vi "Get Linked List Name.vi"(8 "error in (no error)":errorcluster, 10 "Unique ID":string, 11 "Linked List in":refnum<class "Linked List.lvclass">) -> (0 "error out":errorcluster, 1 "I am Root?":bool, 2 "Linked List Name":string, 3 "Linked List out":refnum<class "Linked List.lvclass">)   [LabVIEW 2020, in "Linked Lists.lvlib" / "Linked List.lvclass"]
uses:
  <vilib>/gpm_packages/@cs/linked-list/Source/Linked List/Linked List/Linked List.lvclass
  <vilib>/gpm_packages/@cs/linked-list/Source/Linked List/Linked List Definition/Linked List Definition.lvclass
  <vilib>/gpm_packages/@cs/linked-list/Source/Linked List/Linked List/Linked List.lvclass/Linked List.ctl
  <vilib>/gpm_packages/@cs/lookup-table/Source/LookupTable/LookupTable.lvclass/LookupTable.ctl
  6b1855ba-96a8-42ce-880d-34d98a0d5dd7.vi
  <vilib>/gpm_packages/@cs/lookup-table/Source/LookupTable/Read Table Reference.vi
  6b1855ba-96a8-42ce-880d-34d98a0d5dd7.vi/5a7267ad-595e-4610-9ac2-8bef780848ff.vi
  <vilib>/gpm_packages/@cs/lookup-table/Source/LookupTable/LookupTable.lvclass
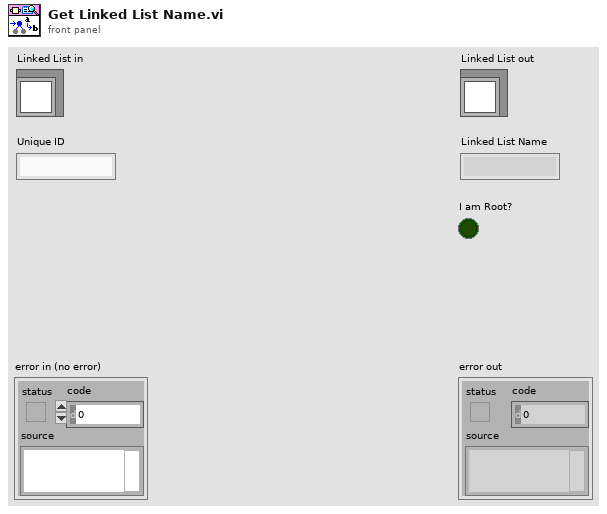
[diagram p1: front panel]
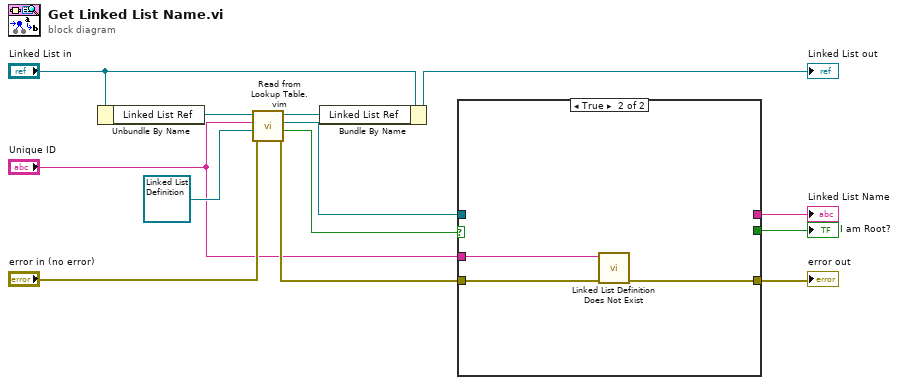
[diagram p0: block diagram]
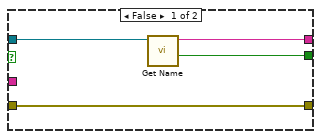
[diagram p2: hidden frame]
diagram:
  n1 = Unbundle By Name("Linked List in") -> ("Linked List Ref"=w13:refnum<data-value>)
  n2 = call "Read from Lookup Table.vim"("error in (no error)"="error in (no error)", "Type"=refnum<class "Linked List Definition.lvclass"> refnum ("Linked List.lvlib:Linked List Definition.lvclass"), "Item Name"="Unique ID", "LookupTable Reference"=w13) -> ("error out"=w5:errorcluster, "Not Found?"=w7:bool, "Value"=w6:refnum<class "Linked List Definition.lvclass">, "LookupTable Reference Out"=w10:refnum<data-value>)  [unwired: 4 in]
  n3 = Bundle By Name(cluster="Linked List in", "Linked List Ref"=w10) -> (→"Linked List out":refnum<class "Linked List.lvclass">)
  n4 = case shown="True" w7 {
    tunnel: w6 -> [w16 _]
    tunnel: w5 -> [w17 w20]
    tunnel: [w17 w19] -> w4
    tunnel: "Unique ID" -> [_ w18]
    tunnel: [w15 _] -> w2
    tunnel: [w14 _] -> w1
    frame False {
      n5 = call <vilib>:"Get Name.vi"("Linked List Definition in"=w16) -> ("I am Root?"=w14:bool, "Name"=w15:string)  [unwired: 8 in, 1 out]
    }
    frame True {
      n6 = call <vilib>:"Linked List Definition Does Not Exist.vi"("Error In"=w20, "Unique ID"=w18) -> ("Error Out"=w19:errorcluster)  [unwired: 9 in]
    }
  }
  "error out" <- w4
  "I am Root?" <- w1
  "Linked List Name" <- w2
